vi "例10.3  利用底层函数采集N幅图像.vi"() -> ()   [LabVIEW 2017]
doc: "The Low-Level Sequence VI acquires a sequence of images and displays the images in an image control using low-level acquisition VIs. A sequence is appropriate for applications in which you want to process multiple images."
uses:
  <vilib>/userdefined/High Color/IMAQdx.ctl
  <vilib>/vision/driver/IMAQdx.llb/IMAQdx Acquisition Mode.ctl
  <vilib>/vision/driver/IMAQdx.llb/IMAQdx Buffer Number Mode.ctl
  <vilib>/vision/driver/NI_Vision_Acquisition_Software.lvlib
panel:
  in  "Camera Name":T1
  out "Image Array":T2[](array[plugin-control])
  in  "Number of Images":u32=5
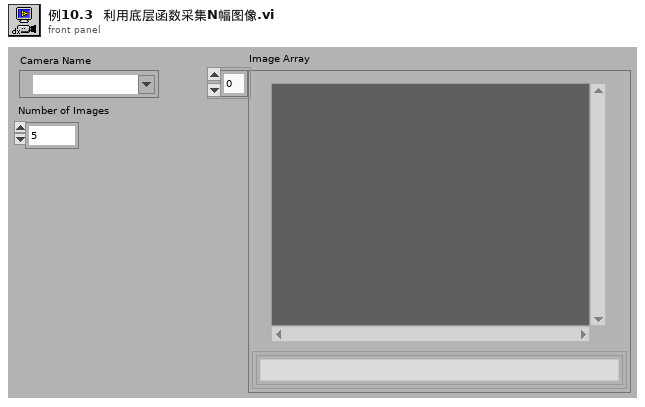
[diagram p1: front panel]
types:
  T1 = typedef "IMAQdx.ctl" = refnum<k21>
  T2 = typedef "IMAQ Image.ctl" = refnum<image>
  T3 = typedef "NI_Vision_Acquisition_Software.lvlib/IMAQdx Acquisition Mode.ctl" = enum32{"One Shot", "Continuous"}
  T4 = typedef "NI_Vision_Acquisition_Software.lvlib/IMAQdx Buffer Number Mode.ctl" = enum32{"Next", "Last", "Buffer Number", "Every", "Last New"}
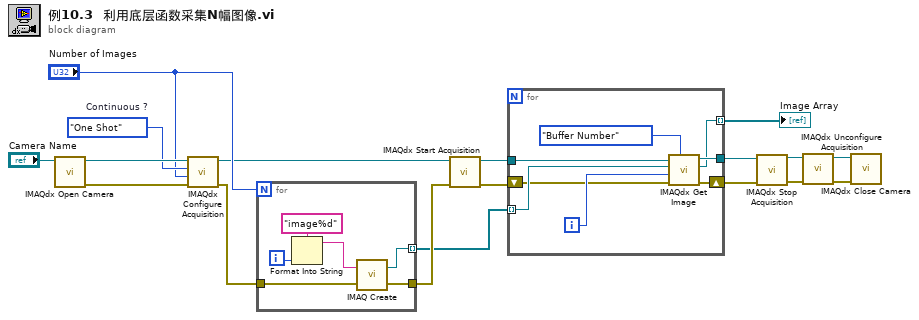
[diagram p0: block diagram]
diagram:
  w15 = IMAQdx_Acquisition_Mode."One Shot"  # Continuous ?
  n1 = call <vilib>:"IMAQdx Open Camera.vi"("Session In"="Camera Name") -> ("error out"=w16:errorcluster, "Session Out"=w17:T1)  [unwired: 2 in, 7 out]
  n2 = call <vilib>:"IMAQdx Configure Acquisition.vi"("error in"=w16, "Number of Buffers"="Number of Images", "Continuous?"=w15, "Session In"=w17) -> ("error out"=w13:errorcluster, "Session Out"=w12:T1)  [unwired: 6 out]
  n3 = for {
    N: "Number of Images" -> [_]
    tunnel: w13 -> [w24]
    tunnel: [w23] -> w9 mode=indexing
    tunnel: [w22] -> w11
    i -> [w21]
    n4 = Format Into String(format string="image%d" ("Image Name"), w21) -> (resulting string=w20:string)  [unwired: 2 in, 1 out]
    n5 = call "IMAQ Create"("Image Name"=w20, "error in (no error)"=w24) -> ("New Image"=w23:T2, "error out"=w22:errorcluster)  [unwired: 2 in, 1 out]
  }
  n6 = call <vilib>:"IMAQdx Start Acquisition.vi"("error in"=w11, "Session In"=w12) -> ("error out"=w8:errorcluster, "Session Out"=w10:T1)  [unwired: 8 out]
  n7 = for {
    tunnel: w9 -> [w31] mode=indexing
    shift-right: [w29] -> w7
    shift-left: w8 -> [w30]
    tunnel: [w28] -> w6
    tunnel: w10 -> [w27]
    tunnel: [w25] -> w1 mode=indexing
    i -> [w32]
    n8 = call <vilib>:"IMAQdx Get Image.vi"("Buffer Number Mode (Next)"=IMAQdx_Buffer_Number_Mode."Buffer Number", "error in"=w30, "Buffer Number In"=w32, "Image In"=w31, "Session In"=w27) -> ("error out"=w29:errorcluster, "Image Out"=w25:T2, "Session Out"=w28:T1)  [unwired: 4 out]
  }
  "Image Array" <- w1
  n9 = call <vilib>:"IMAQdx Stop Acquisition.vi"("error in"=w7, "Session In"=w6) -> ("error out"=w5:errorcluster, "Session Out"=w4:T1)  [unwired: 8 out]
  n10 = call <vilib>:"IMAQdx Unconfigure Acquisition.vi"("error in"=w5, "Session In"=w4) -> ("error out"=w3:errorcluster, "Session Out"=w2:T1)  [unwired: 8 out]
  n11 = call <vilib>:"IMAQdx Close Camera.vi"("error in"=w3, "Session In"=w2) -> ()  [unwired: 10 out]
